vi "writeToXML.vi"(8 "error in (no error)":errorcluster, 10 "ClassLabel":string, 11 "WSSet in":refnum<class "WSSet.lvclass">) -> (0 "error out":errorcluster, 2 "XMLout":string, 3 "WSSet out":refnum<class "WSSet.lvclass">)   [LabVIEW 2014, in "TCSDataDefinitions.lvlib" / "TCSWeatherServerCommand.lvlib" / "WSSet.lvclass"]
uses:
  WSSet.lvclass
  <userlib>/Common/UnitsAndXML/FlattenItemWithUnitToXML/FlattenPressureToXML/PressureUnit.ctl
  <userlib>/Common/UnitsAndXML/FlattenItemWithUnitToXML/FlattenTemperatureAbsToXML/TemperatureAbsUnit.ctl
  WSSet.lvclass/WSSet.ctl
  TCSWeatherServerCommand/TCSWeatherServerCommand.lvclass
  <userlib>/Common/UnitsAndXML/UnitsAndXML.lvlib
  <userlib>/Common/XML/XMLGenerator/XMLGenerator.lvclass
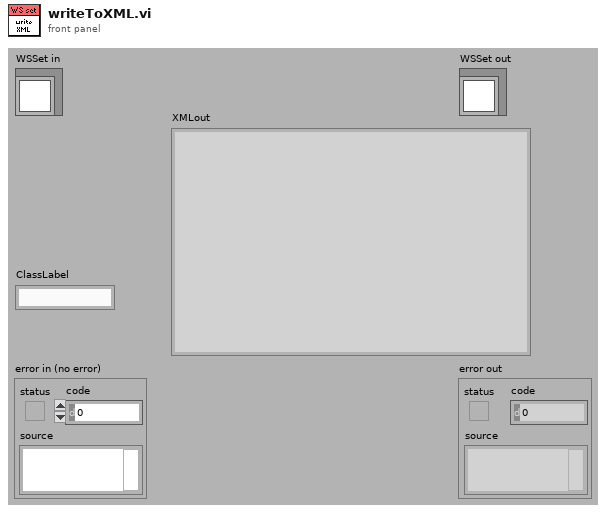
[diagram p1: front panel]
types:
  T1 = typedef "UnitsAndXML.lvlib/TemperatureAbsUnit.ctl" = enum16{"K", "degC", "degF"}
  T2 = typedef "UnitsAndXML.lvlib/PressureUnit.ctl" = enum16{"Pa", "atm", "bar", "mbar", "m.Hg", "psi", "torr"}
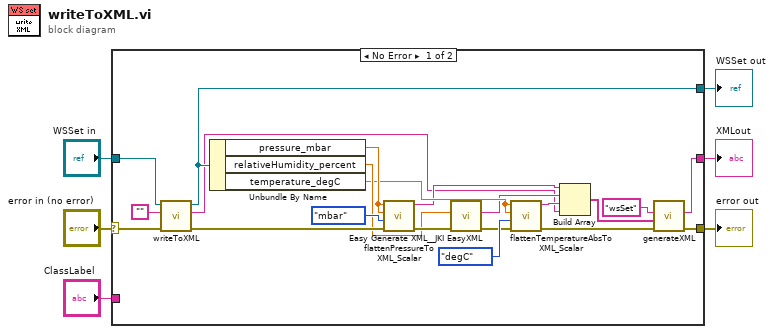
[diagram p0: block diagram]
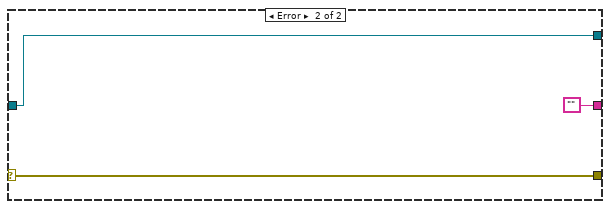
[diagram p2: hidden frame]
diagram:
  n1 = case shown="No Error" "error in (no error)" {
    selector: "error in (no error)" -> [w9 w30]
    tunnel: [w8 w30] -> w5
    tunnel: [w25 w29] -> w3
    tunnel: "WSSet in" -> [w27 w29]
    tunnel: [w10 ""] -> w2
    tunnel: "ClassLabel" -> [_ _]
    frame No Error {
      n2 = call-parent "writeToXML.vi"("error in (no error)"=w9, "ClassLabel"="", "TCSWeatherServerCommand in"=w27) -> ("error out"=w22:errorcluster, "XMLout"=w7:string, "TCSWeatherServerCommand out"=w25:refnum<class "WSSet.lvclass">)  [unwired: 6 in]
      n3 = Unbundle By Name(w25) -> ("pressure_mbar"=w24:dbl[unit], "relativeHumidity_percent"=w20:dbl, "temperature_degC"=w19:dbl[unit])
      n4 = call <userlib>:"flattenPressureToXML_Scalar.vi"("error in (no error)"=w22, "pressureUnitInXML"=PressureUnit."mbar", "pressureAgain"=w24, "pressure"=w24) -> ("error out"=w21:errorcluster, "xmlString"=w16:string)  [unwired: 6 in]
      n5 = call <vilib>:"Easy Generate XML__JKI EasyXML.vi"("error in (no error)"=w21, "LabVIEW Data"=w20) -> ("error out"=w17:errorcluster, "XML String"=w15:string)  [unwired: 8 in]
      n6 = call <userlib>:"flattenTemperatureAbsToXML_Scalar.vi"("error in (no error)"=w17, "temperatureAbsUnitInXML"=TemperatureAbsUnit."degC", "temperatureAbsAgain"=w19, "temperatureAbs"=w19) -> ("error out"=w13:errorcluster, "xmlString"=w14:string)  [unwired: 6 in]
      n7 = Build Array(w16, w15, w14, w7) -> (w12:string[])
      n8 = call <userlib>:"generateXML.vi"("error in"=w13, "childrenXML"=w12, "elementName"="wsSet" ("Class Label")) -> ("error out"=w8:errorcluster, "XML out"=w10:string)  [unwired: 6 in, 1 out]
    }
    frame Error {
    }
  }
  "error out" <- w5
  "WSSet out" <- w3
  "XMLout" <- w2
